vi "Set dt.vi"(8 "error in (no error)":errorcluster, 10 "dt":dbl, 11 "Waveform Buffer in":refnum<class "Waveform Buffer.lvclass">) -> (0 "error out":errorcluster, 3 "Waveform Buffer out":refnum<class "Waveform Buffer.lvclass">)   [LabVIEW 2015, in "Waveform Buffer.lvclass"]
uses:
  Waveform Buffer.lvclass
  Waveform Buffer.lvclass/Waveform Buffer.ctl
  Wfm Segment.ctl
  Data Point.ctl
  DBL Waveform Buffer/DBL Waveform Buffer.lvclass/DBL Waveform Buffer.ctl
  DBL Waveform Buffer/DBL Resize Buffer.vi
  Get Buffer Length.vi
  CDB Waveform Buffer/CDB Waveform Buffer.lvclass
  DBL Waveform Buffer/DBL Waveform Buffer.lvclass
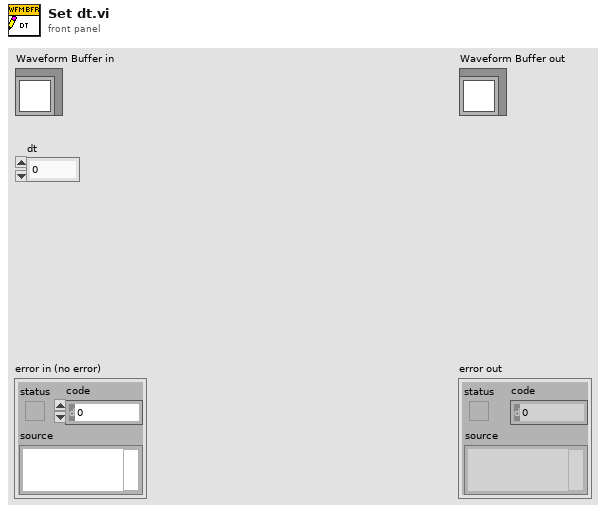
[diagram p1: front panel]
types:
  T1 = typedef "Waveform Buffer.lvclass/Wfm Segment.ctl" = cluster{"ID":u64, "Total samples":i32, "Start":T2, "Finish":T2}
  T2 = typedef "Waveform Buffer.lvclass/Data Point.ctl" = cluster{"Index":i32, "Wfm time":timestamp, "Receive time":timestamp}
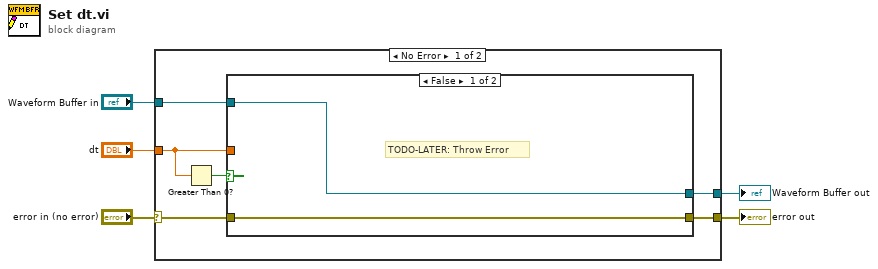
[diagram p0: block diagram]
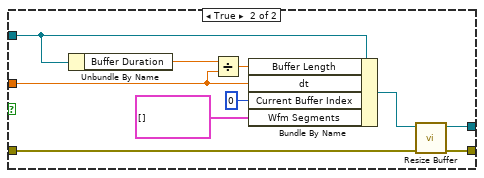
[diagram p2: hidden frame]
diagram:
  n1 = case shown="No Error" "error in (no error)" {
    selector: "error in (no error)" -> [w11 w24]
    tunnel: [w10 w24] -> w4
    tunnel: [w8 w25] -> w2
    tunnel: "Waveform Buffer in" -> [w9 w25]
    tunnel: "dt" -> [w6 _]
    frame No Error {
      n2 = Greater Than 0?(x=w6) -> (x > 0?=w7:bool)
      n3 = case shown="False" w7 {
        tunnel: w11 -> [w13 w23]
        tunnel: [w13 w22] -> w10
        tunnel: w9 -> [w12 w21]
        tunnel: [w12 w16] -> w8
        tunnel: w6 -> [_ w14]
        frame False {
          # "TODO-LATER: Throw Error"
        }
        frame True {
          n4 = Unbundle By Name(w21) -> ("Buffer Duration"=w20:dbl)
          n5 = Divide(x=w20, y=w14) -> (x/y=w19:dbl)
          n6 = Bundle By Name(cluster=w21, "Buffer Length"=w19, "dt"=w14, "Current Buffer Index"=0 ("Current Segment ID"), "Wfm Segments"=T1[] []) -> (w15:refnum<class "Waveform Buffer.lvclass">)
          n7 = call "Resize Buffer.vi"("error in (no error)"=w23, "Waveform Buffer in"=w15) -> ("error out"=w22:errorcluster, "Waveform Buffer out"=w16:refnum<class "Waveform Buffer.lvclass">)  [unwired: 8 in]
        }
      }
    }
    frame Error {
    }
  }
  "error out" <- w4
  "Waveform Buffer out" <- w2
